vi "piezo-cluster-clamp.vi"(2 "cluster carte entree":T3, 3 "cluster carte data":T1) -> (0 "cluster carte sortie":T2, 1 "voltage (V)":dbl)   [LabVIEW 2017]
uses:
  <vilib>/DAQmx/write.llb/DAQmx Write (Analog DBL 1Chan 1Samp).vi
  <vilib>/DAQmx/miscellaneous.llb/DAQmx Fill In Error Info.vi
panel:
  # "SORTIES"
  # "ENTREES"
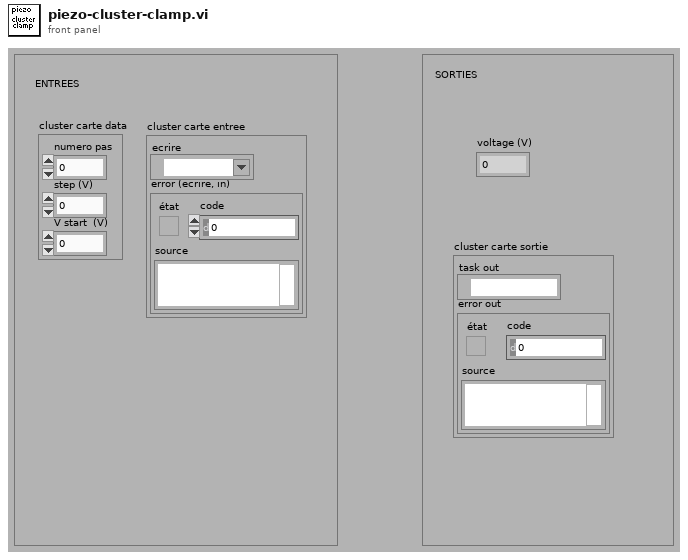
[diagram p1: front panel]
types:
  T1 = cluster{"numero pas":i32, "step (V)":dbl, "V start  (V)":dbl}
  T2 = cluster{"task out":refnum<k21>, "error out":errorcluster}
  T3 = cluster{"ecrire":refnum<k21>, "error (ecrire, in)":errorcluster}
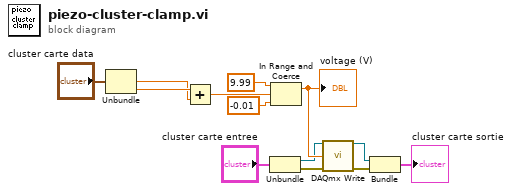
[diagram p0: block diagram]
diagram:
  n1 = Unbundle("cluster carte data") -> ("step (V)"=w1:dbl, "V start  (V)"=w2:dbl)  [unwired: 1 out]
  n2 = Add(x=w2, y=w1) -> (x+y=w10:dbl)
  n3 = Unbundle("cluster carte entree") -> ("ecrire"=w8:refnum<k21>, "error (ecrire, in)"=w7:errorcluster)
  n4 = In Range and Coerce(upper limit=9.99 ("limite haute"), x=w10, lower limit=-0.01 ("limite basse")) -> (coerced(x)=w13:dbl)  [unwired: 1 out]
  "voltage (V)" <- w13
  n5 = call-poly <vilib>:"DAQmx Write.vi"("task/channels in"=w8, "data"=w13, "error in"=w7) -> ("task out"=w6:refnum<k21>, "error out"=w5:errorcluster)  [unwired: 1 in, 10 out]
  n6 = Bundle("task out"=w6, "error out"=w5) -> (→"cluster carte sortie":T2)  [unwired: 1 out]
